vi "Null VVariant Constant__ogtk.vi"() -> (0 "Null VVariant":variant)   [LabVIEW 2023, in "openg_variant.lvlib"]
uses:
  openg_variant.lvlib
panel:
  # "EXPERIMENTAL"
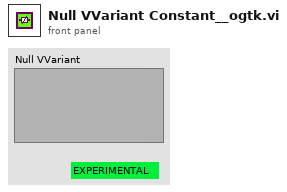
[diagram p1: front panel]
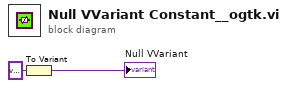
[diagram p0: block diagram]
diagram:
  n1 = To Variant(anything=variant ("variant")) -> (Variant=→"Null VVariant":variant)
